vi "Loader RT Executable Post-Build Action.vi"(5 "Files Generated by Build":path[](array[path]), 6 "Top Level/Always Included VIs":path[](array[path]), 7 "Destination Path":path, 8 "error in (no error)":errorcluster, 9 "Target Name":string, 10 "Build Specification Name":string, 11 "Project Path":path) -> (0 "error out":errorcluster)   [LabVIEW 2021, in "CIF Build Actions.lvlib"]
uses:
  CIF Build Actions.lvlib
  CIFConfigurationFile/typedef/Location Type.ctl
  CIFConfigurationFile/CIF Configuration File Location.vi
  <vilib>/CIF Foundation/CIF Utilities/File/File/Prune to Directory.vi
  <vilib>/Utility/error.llb/Clear Errors.vi
  <vilib>/Utility/libraryn.llb/Check if File or Folder Exists.vi
  <vilib>/regexp/Match Regular Expression.xnode
  <vilib>/CIF Foundation/CIF Utilities/File/File_CIF_U.lvlib
  CIFConfigurationFile/CIF Configuration File.lvlib
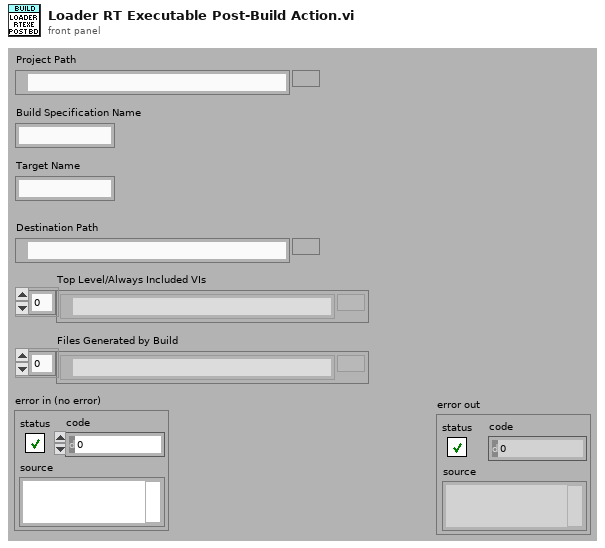
[diagram p1: front panel]
types:
  T1 = typedef "CIF Configuration File.lvlib/Location Type.ctl" = enum16{"Config File", "Manager", "Protos", "Plugins", "UI Plugins", "Logs", "Orchestrations", "Loaders"}
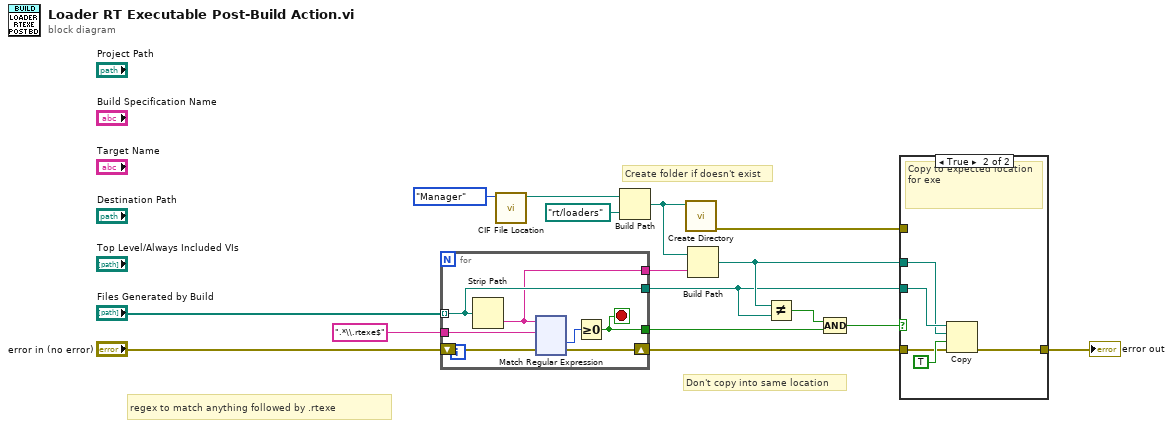
[diagram p0: block diagram]
diagram:
  # "Create folder if doesn't exist"
  # "Don't copy into same location"
  # "regex to match anything followed by .rtexe"
  n1 = for {
    tunnel: "Files Generated by Build" -> [w22] mode=indexing
    tunnel: ".*\\.rtexe$" ("pattern") -> [w23]
    tunnel: [w22] -> w9
    tunnel: [w20] -> w14
    shift-right: [w18] -> w12
    shift-left: "error in (no error)" -> [w19]
    tunnel: [w17] -> w8
    stop <- w17 stop-if-true
    n2 = Strip Path(path=w22) -> (name=w20:string)  [unwired: 1 out]
    n3 = xnode "Match Regular Expression"("input string"=w20, "regular expression"=w23, "error in"=w19) -> ("offset past match"=w21:i32, "error out"=w18:errorcluster)  [unwired: 3 in, 3 out]
    n4 = Greater Or Equal To 0?(x=w21) -> (x >= 0?=w17:bool)
  }
  n5 = call "CIF File Location.vi"("LocationType"=Location_Type."Manager") -> ("Location"=w3:path)  [unwired: 10 in]
  n6 = Build Path(base path=w3, name or relative path=path "rt/loaders") -> (appended path=w2:path)
  n7 = call <vilib>:"Create Directory.vi"("Path In"=w2) -> ("error out"=w5:errorcluster)  [unwired: 9 in, 1 out]
  n8 = Build Path(base path=w2, name or relative path=w14) -> (appended path=w10:path)
  n9 = Not Equal?(x=w10, y=w9) -> (x != y?=w7:bool)
  n10 = Compound Arithmetic op=AND(w7, w8) -> (w6:bool)
  n11 = case shown="True" w6 {
    tunnel: w9 -> [_ w146]
    tunnel: w10 -> [_ w145]
    tunnel: w12 -> [w141 w143]
    tunnel: [w141 w142] -> w11
    tunnel: w5 -> [_ _]
    frame False {
      # "PPL not found, could provide error"
    }
    frame True {
      # "Copy to expected location for exe"
      n12 = Copy(8:w143, 9:TRUE ("overwrite (F)"), 10:w145, 11:w146) -> (0:w142:errorcluster)  [unwired: 1 in, 2 out]
    }
  }
  "error out" <- w11
